vi "MasterSlaveTableDemo.vi"() -> ()   [LabVIEW 2013]
uses:
  TypeDefs/ClickEvent.ctl
  <vilib>/Utility/miscctls.llb/LVPoint32TypeDef.ctl
panel:
  out "Master ClickEvent":T1
  in  "stop":bool
  in  "col span":dbl
  in  "row span":dbl
  in  "col st":dbl
  in  "row st":dbl
  in  "Master Table":string[][](table)
  in  "Slave Table":string[][](table)
  # "The only motivation for splitting the table is that we can make fast slave-wide appearance changes.\nE.g. disabling a row would be a single command (provide all slaves must be disabled). Currently, we have to do it cell by cell\nto preserve the appearance of the master."
  # "What do we lose?\nNot much actually. We'll need to keep track of two table references. The data can easily be combined when sending it to the devices,\nor we can switch to always treating the master separately and just looping over slave devices..."
  # "What challanges are there?\nNeed to link the slave vertical scroll bar to the Master view. (scroll bar control = update table indices!)\nAlso want to be able to shrink the size of the master table in layouts (not only shrinking columns, but resizing the control AND moving the Slave table)..."
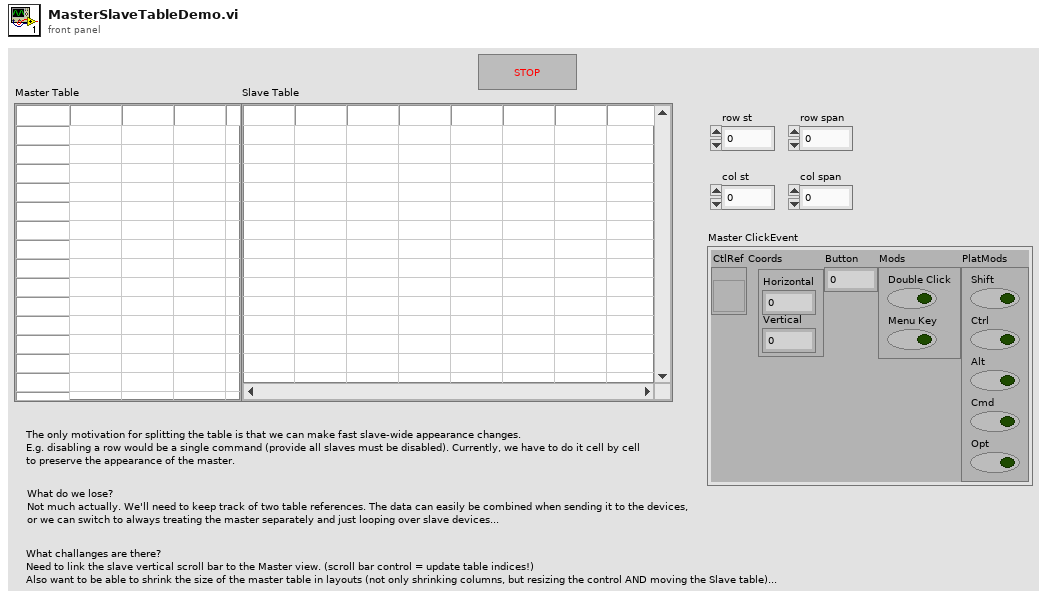
[diagram p1: front panel]
types:
  T1 = typedef "ClickEvent.ctl" = cluster{"CtlRef":refnum<vi>, "Coords":T2, "Button":u16, "Mods":cluster{"Double Click":bool, "Menu Key":bool}, "PlatMods":cluster{"Shift":bool, "Ctrl":bool, "Alt":bool, "Cmd":bool, "Opt":bool}}
  T2 = typedef "LVPoint32TypeDef.ctl" = cluster{"Horizontal":i32, "Vertical":i32}
  T3 = cluster{"Shift":bool, "Ctrl":bool, "Alt":bool, "Cmd":bool, "Opt":bool}
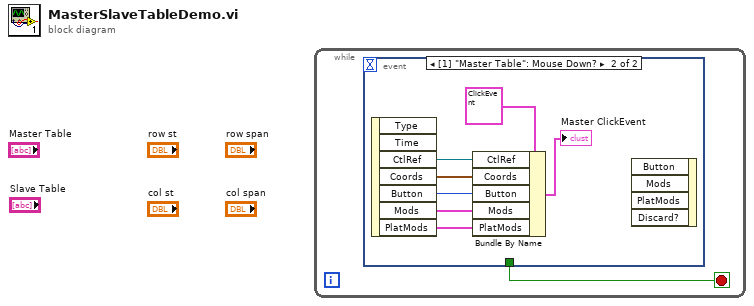
[diagram p0: block diagram]
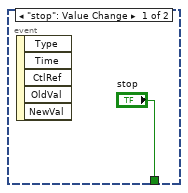
[diagram p2: hidden frame]
diagram:
  n1 = while {
    stop <- w1 stop-if-true
    n2 = event shown="[1] \"Master Table\": Mouse Down?" {
      selector: _ -> [_ _]
      dyn-events: _ -> [_ _]
      timeout: _ -> [_ _]
      tunnel: ["stop" _] -> w1
      event "stop": Value Change {
        n3 = event-data() -> ()  [unwired: 1 in, 5 out]
      }
      event "Master Table": Mouse Down? {
        n4 = event-data() -> ("CtlRef"=w8:refnum<vi>, "Coords"=w7:T2, "Button"=w6:u16, "Mods"=w5:cluster{"Double Click":bool, "Menu Key":bool}, "PlatMods"=w4:T3)  [unwired: 1 in, 2 out]
        n5 = Bundle By Name(cluster=T1 {"CtlRef"=refnum, "Coords"={"Horizontal"=570, "Vertical"=269}, "Button"=1, "Mods"={"Double Click"=TRUE, "Menu Key"=FALSE}, "PlatMods"={"Shift"=FALSE, "Ctrl"=FALSE, "Alt"=FALSE, "Cmd"=FALSE, "Opt"=FALSE}} ("Master ClickEvent"), "CtlRef"=w8, "Coords"=w7, "Button"=w6, "Mods"=w5, "PlatMods"=w4) -> (→"Master ClickEvent":T1)
        n6 = event-data() -> ()  [unwired: 5 in, 1 out]
      }
    }
  }
